vi "Replace Slopes.vi"(8 "error in (no error)":errorcluster, 11 "Maze in":refnum<class "Maze.lvclass">) -> (0 "error out":errorcluster, 3 "Maze out":refnum<class "Maze.lvclass">)   [LabVIEW 2021, in "Maze.lvclass"]
uses:
  Maze.lvclass
  Maze.lvclass/Maze.ctl
panel:
  out "Maze 2":string[][](array[string])
  out "Maze":string[][](array[string])
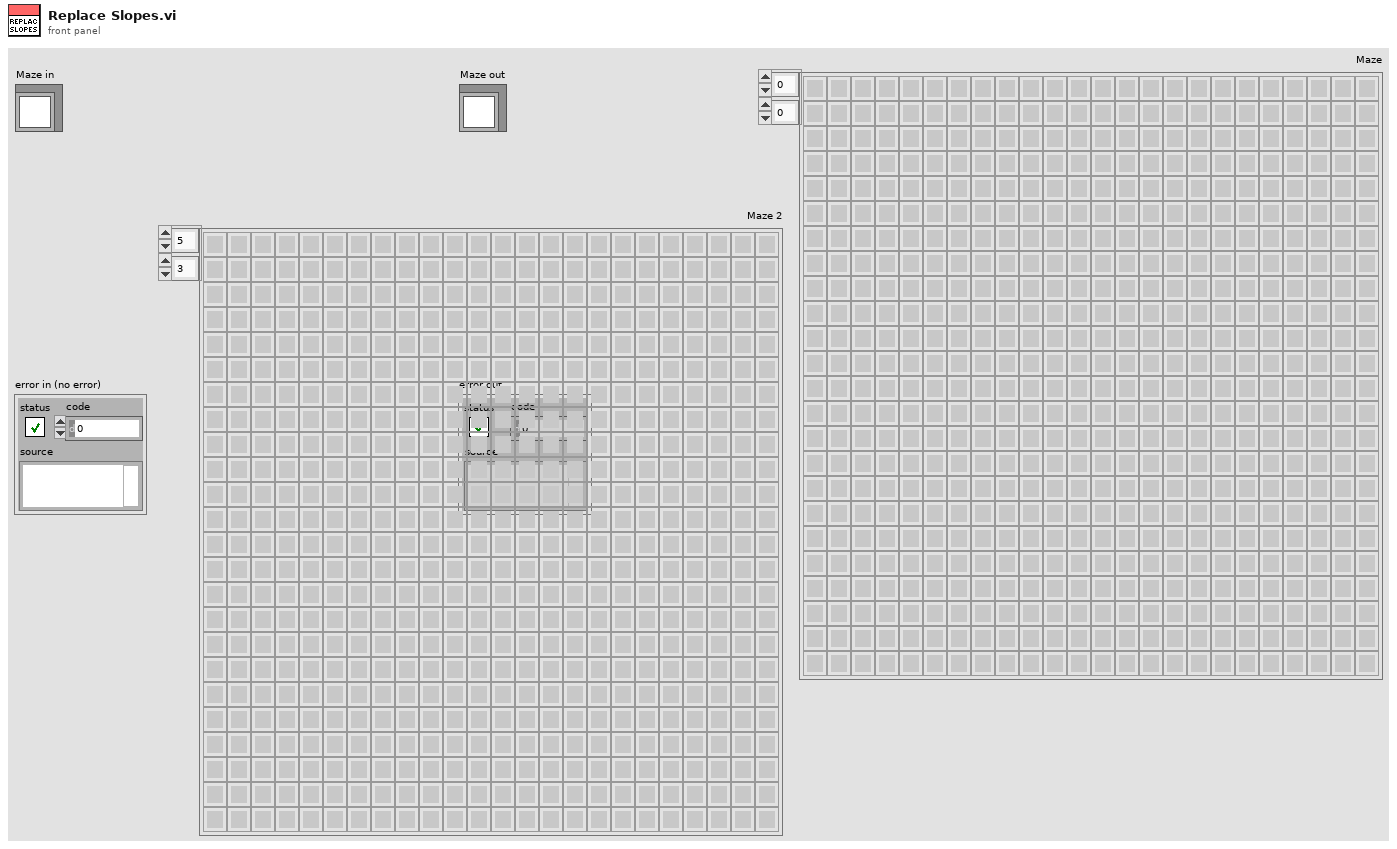
[diagram p1: front panel]
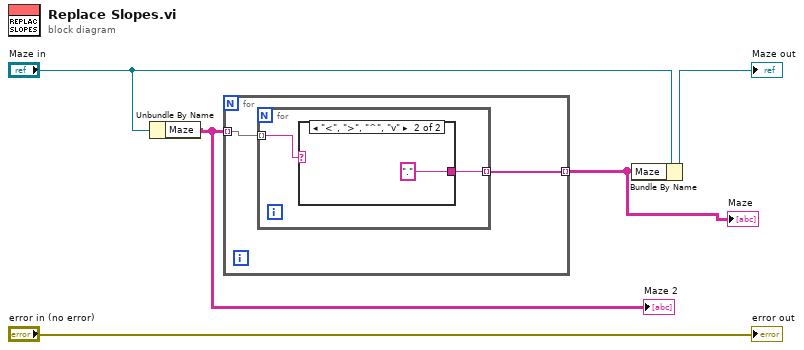
[diagram p0: block diagram]
diagram:
  n1 = Unbundle By Name("Maze in") -> ("Maze"=w1:string[][])
  "Maze 2" <- w1
  n2 = for {
    tunnel: w1 -> [w7] mode=indexing
    tunnel: [w6] -> w2 mode=indexing
    n3 = for {
      tunnel: w7 -> [w9] mode=indexing
      tunnel: [w8] -> w6 mode=indexing
      n4 = case shown="\"<\", \">\", \"^\", \"v\"" w9 {
        selector: w9 -> [w10 _]
        tunnel: [w10 "."] -> w8
        frame Default {
        }
        frame "<", ">", "^", "v" {
        }
      }
    }
  }
  "Maze" <- w2
  n5 = Bundle By Name(cluster="Maze in", "Maze"=w2) -> (→"Maze out":refnum<class "Maze.lvclass">)
  "error out" <- "error in (no error)"
